vi "Write Switch Channel.vi"(8 "error in (no error)":errorcluster, 10 "Digitizer Channel Setting":T1={"Connection"="None"}, 11 "Switch Channel configuration":refnum<class "Switch Channel configuration.lvclass">) -> (0 "error out":errorcluster, 3 "Switch Channel configuration out":refnum<class "Switch Channel configuration.lvclass">)   [LabVIEW 2025, in "Switch.lvlib" / "Switch Channel configuration.lvclass"]
uses:
  Switch Channel configuration.lvclass
  Switch Channel Setting.ctl
  Switch Channel configuration.lvclass/Switch Channel configuration.ctl
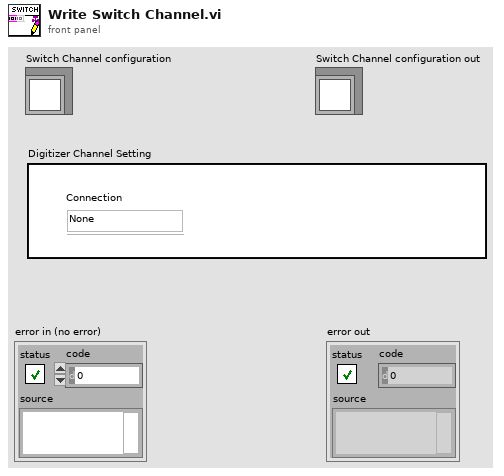
[diagram p1: front panel]
types:
  T1 = typedef "Switch.lvlib/Switch Channel configuration.lvclass/Switch Channel Setting.ctl" = cluster{"Connection":string}
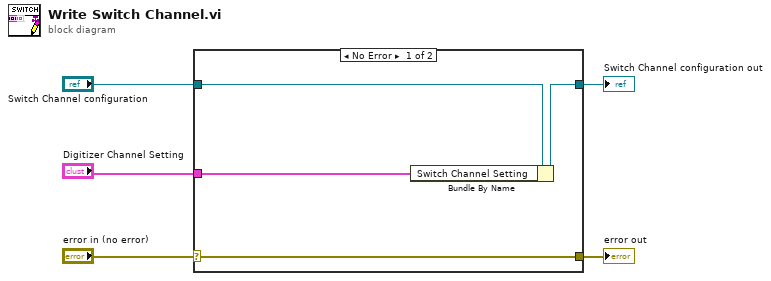
[diagram p0: block diagram]
diagram:
  n1 = case shown="No Error" "error in (no error)" {
    selector: "error in (no error)" -> [w9 w10]
    tunnel: [w9 w10] -> w4
    tunnel: [w7 w11] -> w2
    tunnel: "Switch Channel configuration" -> [w8 w11]
    tunnel: "Digitizer Channel Setting" -> [w6 _]
    frame No Error {
      n2 = Bundle By Name(cluster=w8, "Switch Channel Setting"=w6) -> (w7:refnum<class "Switch Channel configuration.lvclass">)
    }
    frame Error {
    }
  }
  "error out" <- w4
  "Switch Channel configuration out" <- w2
